vi "Analysis GUI.vi"(11 "Parameters":T1={"Results Path"=path "C:/testdata/Logs", "Temp Path"=path "C:/testdata/Temp", "Remote Path"=path "d:/testdata/Logs", "Analysis VIs"=[path "C:/addons/TestStand Examples for HIL/Continuous Monitoring Tester/Sequences/Analysis/Builds/TestStand Analysis Steps.lvlibp/Post Process Analysis Steps/Analysis.LevelTransition.vi"], "Report Passed?"=FALSE, "Group Channels?"=FALSE}) -> ()   [LabVIEW 2015, in "NIAnalysis.lvlib"]
uses:
  NIAnalysis.lvlib
  Types/AnalysisGUI.Parameters.ctl
  Types/AnalysisGUI.Refs.ctl
panel:
  out "Cycle":i32
  in  "error in (no error)":errorcluster
  in  "Stop":bool
  out "Results Directory":path=path "d:/testdata/TestResults"
  in  "Results":string(tree)
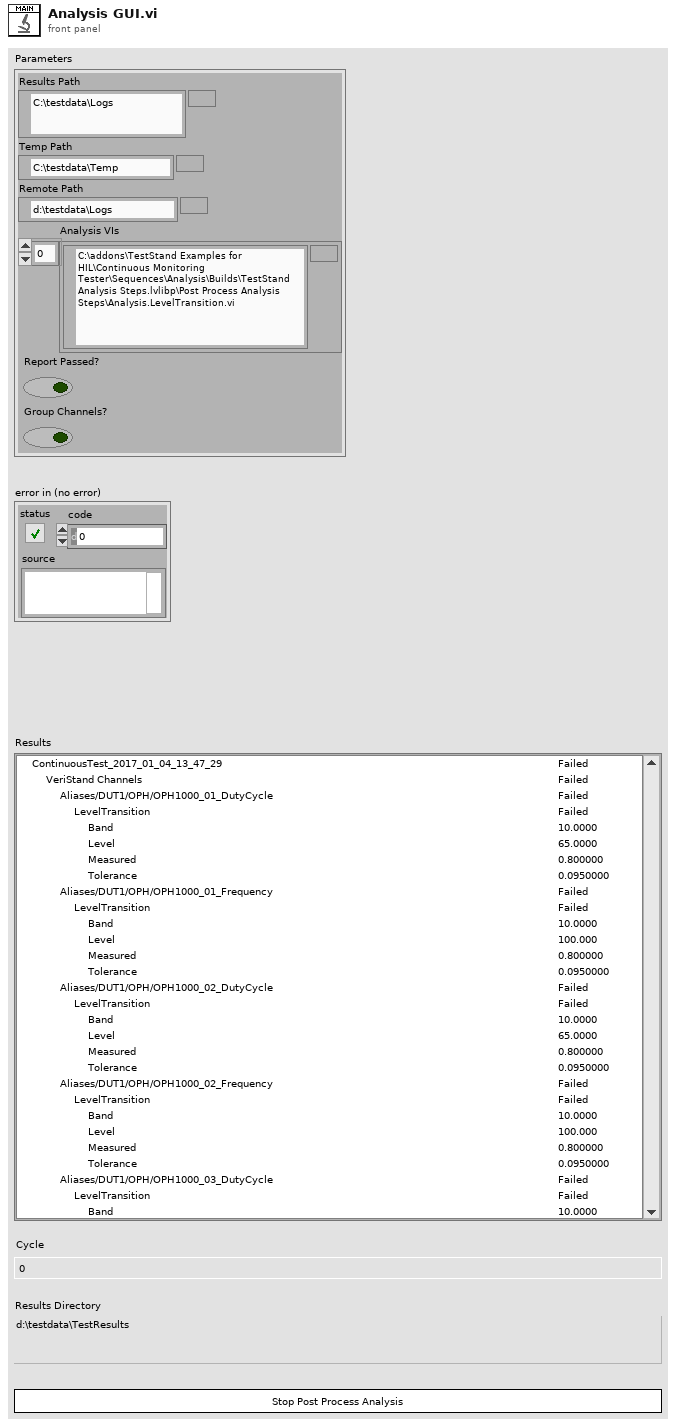
[diagram p1: front panel]
types:
  T1 = typedef "NIAnalysis.lvlib/AnalysisGUI.Parameters.ctl" = cluster{"Results Path":path, "Temp Path":path, "Remote Path":path, "Analysis VIs":path[], "Report Passed?":bool, "Group Channels?":bool}
  T2 = typedef "NIAnalysis.lvlib/AnalysisGUI.Refs.ctl" = cluster{"Cycle":refnum<vi>, "Tree":refnum<vi>, " VI":refnum<vi>}
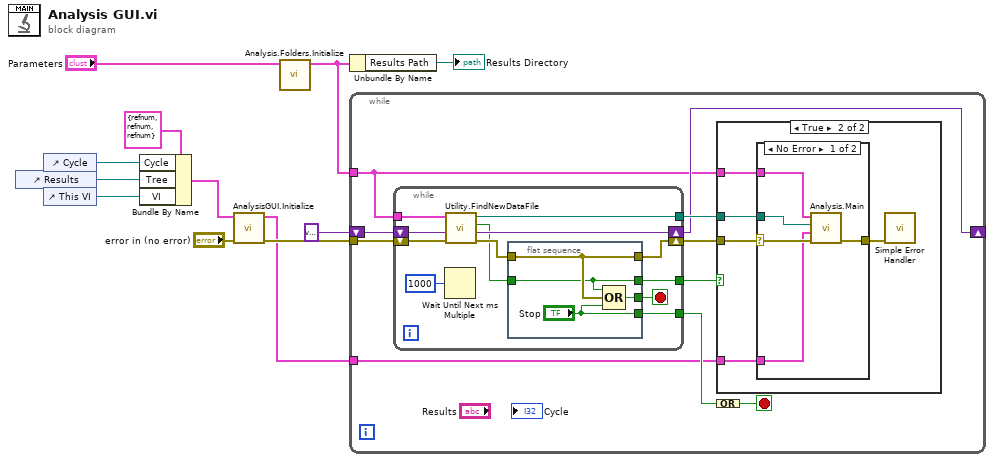
[diagram p0: block diagram]
diagram:
  n1 = control-ref of="Results"() -> (w9:refnum<vi>)
  n2 = control-ref of="Cycle"() -> (w7:refnum<vi>)
  n3 = control-ref of="This VI"() -> (w4:refnum<vi>)
  n4 = Bundle By Name(cluster=T2 {"Cycle"=refnum, "Tree"=refnum, " VI"=refnum} ("output cluster"), "Cycle"=w7, "Tree"=w9, "VI"=w4) -> (w10:T2)
  n5 = call "AnalysisGUI.Initialize.vi"("error in (no error)"="error in (no error)", "Refs"=w10) -> ("error out"=w12:errorcluster, "Refs"=w6:T2)  [unwired: 8 in]
  n6 = call "Analysis.Folders.Initialize.vi"("Parameters in"="Parameters") -> ("Parameters out"=w1:T1)  [unwired: 10 in]
  n7 = Unbundle By Name(w1) -> ("Results Path"=→"Results Directory":path)
  n8 = while {
    tunnel: w12 -> [w20]
    tunnel: w6 -> [w19]
    shift-right: [w16] -> _
    shift-left: variant -> [w17]
    tunnel: w1 -> [w13]
    stop <- w21 stop-if-true
    n9 = while {
      shift-right: [w43] -> w15
      shift-left: w20 -> [w45]
      tunnel: [w36] -> w18
      tunnel: [w42] -> w14
      tunnel: [w40] -> w22
      shift-right: [w38] -> w16
      shift-left: w17 -> [w39]
      tunnel: w13 -> [w35]
      stop <- w41 stop-if-true
      n10 = Wait Until Next ms Multiple(millisecond multiple=u32 1000) -> ()  [unwired: 1 out]
      n11 = call "Utility.FindNewDataFile.vi"("error in (no error)"=w45, "LookupTable"=w39, "Parameters"=w35) -> ("error out"=w44:errorcluster, "LookupTable out"=w38:variant, "Found"=w37:bool, "Data Path"=w36:path)  [unwired: 5 in]
      n12 = flat-sequence {
        tunnel: w37 -> [w46]
        tunnel: [w49] -> w41
        tunnel: w44 -> [w48]
        tunnel: [w48] -> w43
        tunnel: [w46] -> w42
        tunnel: ["Stop"] -> w40
        frame #0 {
          n13 = Compound Arithmetic op=OR(w46, w48, "Stop") -> (w49:bool)
        }
      }
    }
    n14 = case shown="True" w14 {
      tunnel: w13 -> [_ w27]
      tunnel: w19 -> [_ w25]
      tunnel: w18 -> [_ w26]
      tunnel: w15 -> [_ w23]
      frame False {
      }
      frame True {
        n15 = case shown="No Error" w23 {
          selector: w23 -> [w32 w33]
          tunnel: w26 -> [w30 _]
          tunnel: w27 -> [w31 _]
          tunnel: w25 -> [w28 _]
          tunnel: [w29 w33] -> w24
          frame No Error {
            n16 = call "Analysis.Main.vi"("error in (no error)"=w32, "Refs"=w28, "Data Path"=w30, "Parameters"=w31) -> ("error out"=w29:errorcluster)  [unwired: 6 in, 1 out]
          }
          frame Error {
          }
        }
        n17 = call <vilib>:"Simple Error Handler.vi"("error in (no error)"=w24) -> ()  [unwired: 4 in, 5 out]
      }
    }
    n18 = Compound Arithmetic op=OR(w22) -> (w21:bool)
  }
